vi "instr.DSO_Data.vi"(7 "Timeout(ms)":u32=600, 8 "错误输入（无错误）":errorcluster={"status"=FALSE, "code"=-1073807339, "source"="Agilent.DSO.vi->new display API.DSO2002A.vi中的VISA读取"}, 10 "CMD write":string=":WAVeform:DATA?", 11 "VISA.in":refnum<visa-resource-name>="USB0::0x0957::0x179B::MY52014069::INSTR") -> (0 "错误输出":errorcluster={"status"=FALSE, "code"=1073676294, "source"="Agilent.DSO.vi->new display API.DSO2002A.vi中的VISA读取"}, 1 "Reply info":string="#800000500~~~|||{zzyyyxxwwvvvvvuuuuuuuuvwwwwwxxxxzz{{|}}~~~~}}|{{{zyyxxwwwvvvvuvuuuuvvuuvwvwxxxxxyzz{||}}~~~}}|{{{zyyxxxwwwvvvvuvuuuuvuvvvvwwxxyyyyz{||}~~~~}}|{{{zyyxxxwvvvvvvvuvuuuuuvvvwwwxxxyyz{{{|}}~~~}}||{zzyyyxxwwwvvvvuuuuuvuvvvvvwwwxxyyzz{{|}~\n", 2 "Value":dbl, 3 "VISA.out":refnum<visa-resource-name>="USB0::0x0957::0x179B::MY52014069::INSTR")   [LabVIEW 2012, in "Lib_UEL.ATE.lvlib" / "Lib_Instrument.lvlib"]
uses:
  Lib_Instrument.lvlib
panel:
  # ":TRIG:EDGE:COUP  AC|DC"
  # ":SINGLE|RUN|STOP"
  # ":CHAN1:PROB 1"
  # "*RST"
  # ":CHAN1:COUP AC|DC"
  # ":CHAN1:SCAL   unit:v"
  # ":TIM:SCAL     unit:S"
  # ":MEAS:VPP|VMAX|VRMS|FREQ?"
  # ":TRIG:EDGE:LEV  unit:v"
  # ":TRIG:MODE  EDGE"
  # "DSO2002X"
  # "DSO1002X"
  # ":TRIG:SWE AUTO|NORMAL"
  # ":TRIG:EDGE:SWE AUTO|NORMAL"
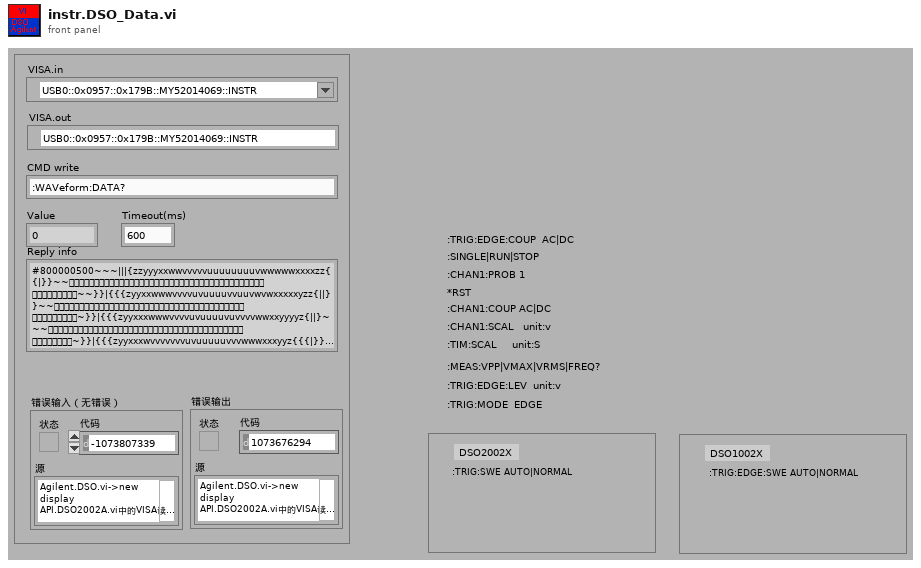
[diagram p1: front panel]
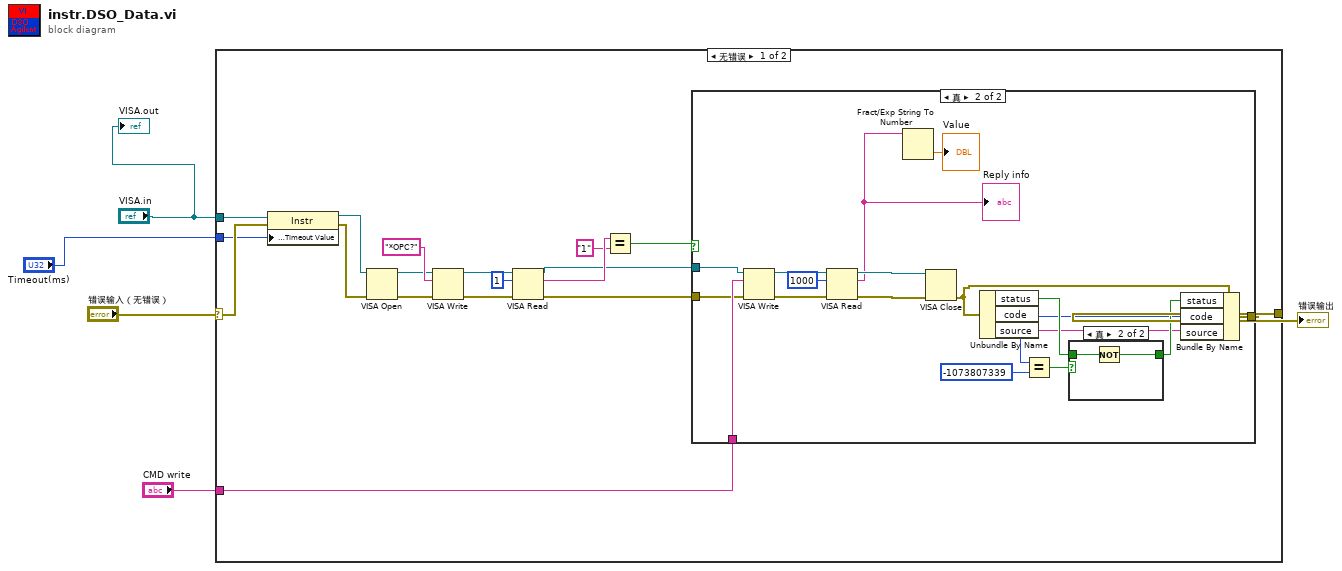
[diagram p0: block diagram]
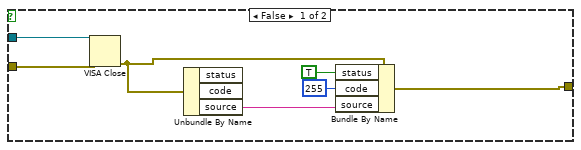
[diagram p2: hidden frame]
diagram:
  n1 = case shown="无错误" "错误输入（无错误）" {
    selector: "错误输入（无错误）" -> [w8 w52]
    tunnel: "CMD write" -> [w23 _]
    tunnel: "VISA.in" -> [w10 _]
    tunnel: [w22 w52] -> w4
    tunnel: "Timeout(ms)" -> [w6 _]
    frame No Error {
      n2 = property class="Instr"(reference=w10, error in=w8, "General Settings:Timeout Value"=w6) -> (reference out=w9:refnum<visa-resource-name>, error out=w7:errorcluster)
      n3 = VISA Open(error in (no error)=w7, VISA resource name=w9) -> (VISA resource name=w11:refnum<visa-resource-name>, error out=w21:errorcluster)  [unwired: 3 in]
      n4 = VISA Write(VISA resource name=w11, write buffer="*OPC?" ("写入缓冲区"), error in (no error)=w21) -> (VISA resource name out=w20:refnum<visa-resource-name>, error out=w19:errorcluster)  [unwired: 1 out]
      n5 = VISA Read(VISA resource name=w20, byte count=u32 1 ("字节总数"), error in (no error)=w19) -> (VISA resource name out=w14:refnum<visa-resource-name>, read buffer=w16:string, error out=w13:errorcluster)  [unwired: 1 out]
      n6 = Equal?(x=w16, y="1") -> (x = y?=w12:bool)
      n7 = case shown="真" w12 {
        tunnel: w23 -> [_ w44]
        tunnel: [w24 w33] -> w22
        tunnel: w14 -> [w30 w32]
        tunnel: w13 -> [w29 w31]
        frame False {
          n8 = VISA Close(VISA resource name=w30, error in (no error)=w29) -> (error out=w28:errorcluster)
          n9 = Unbundle By Name(w28) -> ("source"=w25:string)  [unwired: 2 out]
          n10 = Bundle By Name(cluster=w28, "status"=TRUE, "code"=255, "source"=w25) -> (w24:errorcluster)
        }
        frame True {
          n11 = VISA Write(VISA resource name=w32, write buffer=w44, error in (no error)=w31) -> (VISA resource name out=w45:refnum<visa-resource-name>, error out=w46:errorcluster)  [unwired: 1 out]
          n12 = VISA Read(VISA resource name=w45, byte count=u32 1000 ("字节总数"), error in (no error)=w46) -> (VISA resource name out=w47:refnum<visa-resource-name>, read buffer=w42:string, error out=w48:errorcluster)  [unwired: 1 out]
          "Reply info" <- w42
          n13 = Fract/Exp String To Number(string=w42) -> (number=→"Value":dbl)  [unwired: 3 in, 1 out]
          n14 = VISA Close(VISA resource name=w47, error in (no error)=w48) -> (error out=w37:errorcluster)
          n15 = Unbundle By Name(w37) -> ("status"=w38:bool, "code"=w35:i32, "source"=w34:string)
          n16 = Equal?(x=w35, y=-1073807339) -> (x = y?=w39:bool)
          n17 = case shown="真" w39 {
            tunnel: w38 -> [w49 w51]
            tunnel: [w49 w50] -> w36
            frame False {
            }
            frame True {
              n18 = Not(x=w51) -> (.not. x?=w50:bool)
            }
          }
          n19 = Bundle By Name(cluster=w37, "status"=w36, "code"=w35, "source"=w34) -> (w33:errorcluster)
        }
      }
    }
    frame Error {
    }
  }
  "错误输出" <- w4
  "VISA.out" <- "VISA.in"
